vi "Example FlatSequence 1.vi"() -> ()   [LabVIEW 2014]
panel:
  out "time (ms)":i32
  out "Error Out":errorcluster
  in  "Error In":errorcluster
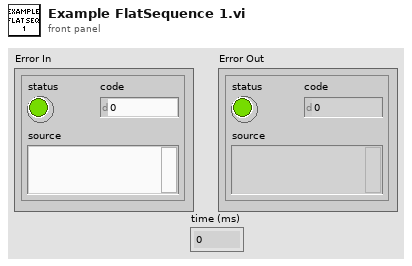
[diagram p1: front panel]
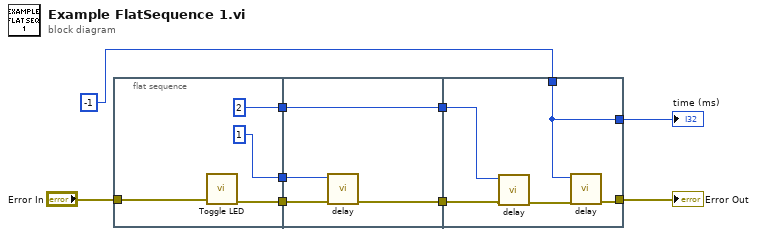
[diagram p0: block diagram]
diagram:
  n1 = flat-sequence {
    tunnel: "Error In" -> [w13]
    tunnel: [w12] -> w7
    tunnel: [1 ("time (ms)")] -> w5
    tunnel: [2 ("time (ms)")] -> w3
    tunnel: w7 -> [w17]
    tunnel: [w16] -> w6
    tunnel: w5 -> [w15]
    tunnel: [w14] -> w4
    tunnel: w3 -> [w14]
    tunnel: [w19] -> w9
    tunnel: w6 -> [w22]
    tunnel: w4 -> [w21]
    tunnel: -1 ("time (ms)") -> [w18]
    tunnel: [w18] -> w1
    frame #0 {
      n2 = call "Toggle LED.vi"("Error In"=w13) -> ("Error Out"=w12:errorcluster)  [unwired: 10 in]
    }
    frame #1 {
      n3 = call "delay.vi"("Error In"=w17, "time (ms)"=w15) -> ("Error Out"=w16:errorcluster)  [unwired: 9 in]
    }
    frame #2 {
      n4 = call "delay.vi"("Error In"=w22, "time (ms)"=w21) -> ("Error Out"=w20:errorcluster)  [unwired: 9 in]
      n5 = call "delay.vi"("Error In"=w20, "time (ms)"=w18) -> ("Error Out"=w19:errorcluster)  [unwired: 9 in]
    }
  }
  "Error Out" <- w9
  "time (ms)" <- w1
